vi "Teleop_Calc_Fly_R.vi"(11 "Teleop Local Data in":T1) -> (3 "Teleop Local Data out":T1)   [LabVIEW 2016]
uses:
  Typedefs/typedef_cluster_Teleop Local Data.ctl
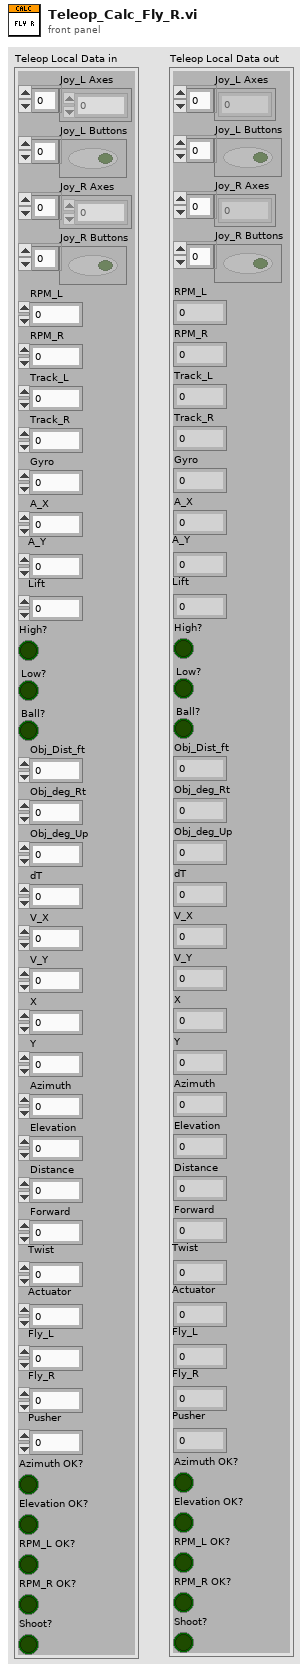
[diagram p1: front panel]
types:
  T1 = typedef "typedef_cluster_Teleop Local Data.ctl" = cluster{"Joy_L Axes":dbl[], "Joy_L Buttons":bool[], "Joy_R Axes":dbl[], "Joy_R Buttons":bool[], "RPM_L":dbl, "RPM_R":dbl, "Track_L":dbl, "Track_R":dbl, "Gyro":dbl, "A_X":dbl, "A_Y":dbl, "Lift":dbl, "High?":bool, "Low?":bool, "Ball?":bool, "Obj_Dist_ft":dbl, "Obj_deg_Rt":dbl, "Obj_deg_Up":dbl, "dT":dbl, "V_X":dbl, "V_Y":dbl, "X":dbl, "Y":dbl, "Azimuth":dbl, "Elevation":dbl, "Distance":dbl, "Forward":dbl, "Twist":dbl, "Actuator":dbl, "Fly_L":dbl, "Fly_R":dbl, "Pusher":dbl, "Azimuth OK?":bool, "Elevation OK?":bool, "RPM_L OK?":bool, "RPM_R OK?":bool, "Shoot?":bool}
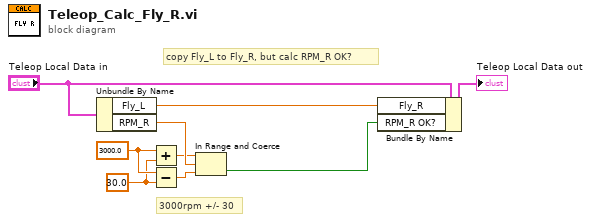
[diagram p0: block diagram]
diagram:
  w5 = 30.0 ("upper limit")
  w6 = 3000.0 ("upper limit")
  # "copy Fly_L to Fly_R, but calc RPM_R OK?"
  # "3000rpm +/- 30"
  n1 = Unbundle By Name("Teleop Local Data in") -> ("Fly_L"=w2:dbl, "RPM_R"=w7:dbl)
  n2 = Add(x=w6, y=w5) -> (x+y=w4:dbl)
  n3 = Subtract(x=w6, y=w5) -> (x-y=w3:dbl)
  n4 = In Range and Coerce(upper limit=w4, x=w7, lower limit=w3) -> (In Range?=w1:bool)  [unwired: 1 out]
  n5 = Bundle By Name(cluster="Teleop Local Data in", "Fly_R"=w2, "RPM_R OK?"=w1) -> (→"Teleop Local Data out":T1)
